vi "qOAD.vi"(0 "System no.":i32=1 min=1 max=4 step=1, 2 "Channel to query":string[](array[string]), 3 "All channels?":bool, 4 "Channel identifier?":bool=TRUE, 5 "error in":errorcluster) -> (14 "Driving voltage":dbl[](array[numeric]) format="%.6f", 19 "error out":errorcluster)   [LabVIEW 2026]
doc: "Returns last commanded open loop Analog Driving voltage of given PiezoWalk channels.\n\nE-755, E-861, E-872: If All channels? = TRUE, then Channel identifier? must be FALSE"
panel:
  # "Returns last commanded open loop Analog Driving voltage of \ngiven PiezoWalk channels."
  # "If all channels: use"
  # "Query"
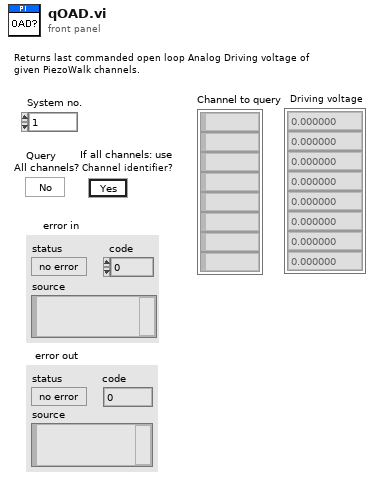
[diagram p1: front panel]
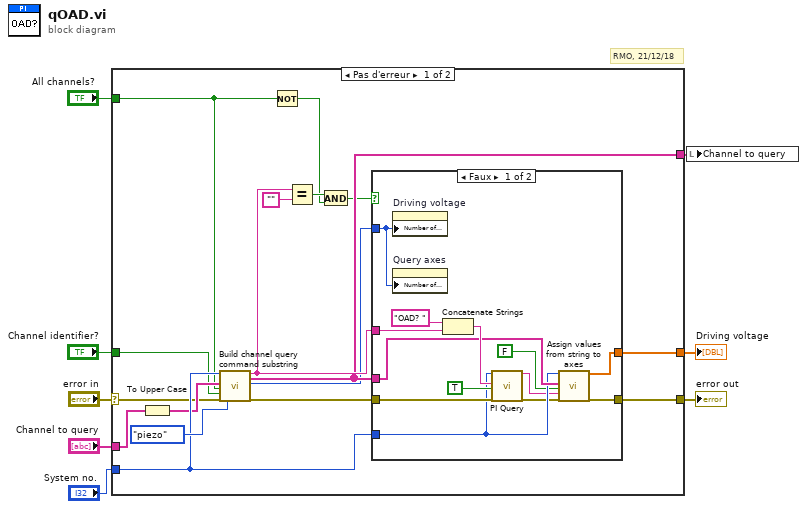
[diagram p0: block diagram]
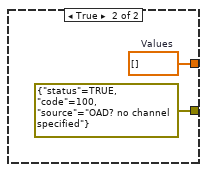
[diagram p2: hidden frame]
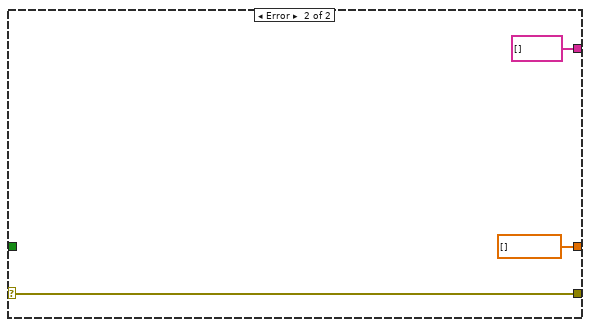
[diagram p3: hidden frame]
diagram:
  # "RMO, 21/12/18"
  n1 = case shown="Pas d'erreur" "error in" {
    selector: "error in" -> [w9 w41]
    tunnel: [w25 dbl[] [] ("Values")] -> w8
    tunnel: "Channel to query" -> [w24 _]
    tunnel: [w11 w41] -> w6
    tunnel: "Channel identifier?" -> [w12 _]
    tunnel: "System no." -> [w15 _]
    tunnel: [w17 string[] [] ("Axes to query out")] -> w3
    tunnel: "All channels?" -> [w13 _]
    frame No Error {
      n2 = To Upper Case(1:w24) -> (0:w14:string[])
      n3 = call "Build channel query command substring.vi"("System no."=w15, "Channels to query in"=w14, "Query\nAll channels?"=w13, "For all channels: use\nChannel identifier?"=w12, "error in"=w9, "Channel type"=enum16{"piezo", "sensor"}."piezo") -> ("Command substring"=w18:string, "Channels to query out"=w17:string[], "Number of rows"=w16:u32, "error out"=w19:errorcluster)  [unwired: 1 in, 9 out]
      n4 = Not(x=w13) -> (.not. x?=w21:bool)
      n5 = Equal?(x=w18, y="" ("x")) -> (x = y?=w22:bool)
      n6 = And(x=w22, y=w21) -> (x .and. y?=w10:bool)
      n7 = case shown="Faux" w10 {
        tunnel: [w35 w39] -> w25
        tunnel: w19 -> [w34 _]
        tunnel: w18 -> [w33 _]
        tunnel: w17 -> [w32 _]
        tunnel: w16 -> [w31 _]
        tunnel: w15 -> [w30 _]
        tunnel: [w28 errorcluster {"status"=TRUE, "code"=100, "source"="OAD? no channel specified"} ("error out")] -> w11
        frame False {
          n8 = property on="Driving voltage" class="Tabl (strict)"("Number of Rows"=w31) -> ()  [unwired: 2 in, 2 out]
          n9 = property on="Query axes" class="Tabl (strict)"("Number of Rows"=w31) -> ()  [unwired: 2 in, 2 out]
          n10 = Concatenate Strings("OAD? ", w33) -> (w36:string)
          n11 = call "PI Query.vi"("System no."=w30, "String to send"=w36, "Attach termination char.?"=TRUE ("Attach Linefeed?"), "error in"=w34) -> ("String read"=w26:string, "error out"=w27:errorcluster)  [unwired: 3 in, 11 out]
          n12 = call "Assign values from string to axes.vi"("System no."=w30, "Queried axes"=w32, "All axes queried?"=FALSE, "Input String"=w26, "error in"=w27) -> ("Values"=w35:dbl[], "error out"=w28:errorcluster)  [unwired: 4 in, 9 out]
        }
        frame True {
          w39 = dbl[] []  # Values
        }
      }
    }
    frame Error {
    }
  }
  "error out" <- w6
  "Driving voltage" <- w8
  n13 = local write "Channel to query"(w3) -> ()
